vi "Read Unsaved changes.vi"(11 "ConfigManager.Text in":refnum<class "ConfigManager.Text.lvclass">) -> (2 "Unsaved changes":string[](array[string]), 3 "ConfigManager.Text out":refnum<class "ConfigManager.Text.lvclass">)   [LabVIEW 2013, in "CfgManager.Text.lvlib" / "ConfigManager.Text.lvclass"]
uses:
  ConfigManager.Text.lvclass
  ConfigManager.Text.lvclass/ConfigManager.Text.ctl
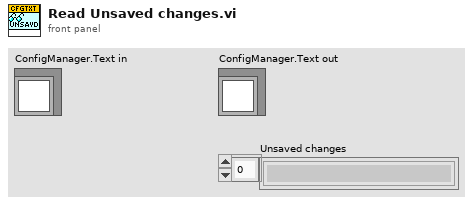
[diagram p1: front panel]
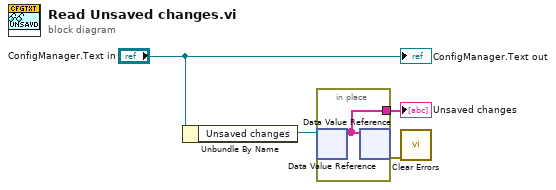
[diagram p0: block diagram]
diagram:
  n1 = Unbundle By Name("ConfigManager.Text in") -> ("Unsaved changes"=w3:refnum<data-value>)
  n2 = in-place {
    in-place-border: [w5] -> w2
    n3 = in-place-dvr #1(w3) -> (w5:string[])  [unwired: 1 out]
    n4 = in-place-dvr #1(w5) -> (w1:errorcluster)  [unwired: 1 out]
  }
  "Unsaved changes" <- w2
  n5 = call <vilib>:"Clear Errors.vi"("error in (no error)"=w1) -> ()  [unwired: 6 in, 1 out]
  "ConfigManager.Text out" <- "ConfigManager.Text in"
